vi "DSF.Engine.Framework.Active Plugins.vi"(8 "error in (no error)":errorcluster, 11 "Framework in":refnum<class "Framework.lvclass">) -> (0 "error out":errorcluster, 2 "active Plugin indices":i32[](array[numeric]), 3 "Framework out":refnum<class "Framework.lvclass">)   [LabVIEW 2016, in "DSF.Engine.lvlib" / "Framework.lvclass"]
uses:
  Framework.lvclass
  Framework.lvclass/Framework.ctl
  Plugin/Plugin.lvclass/Plugin.ctl
  Shared/Classes/Timing/DSF.Shared.Timing.lvclass
  Plugin/Plugin.lvclass
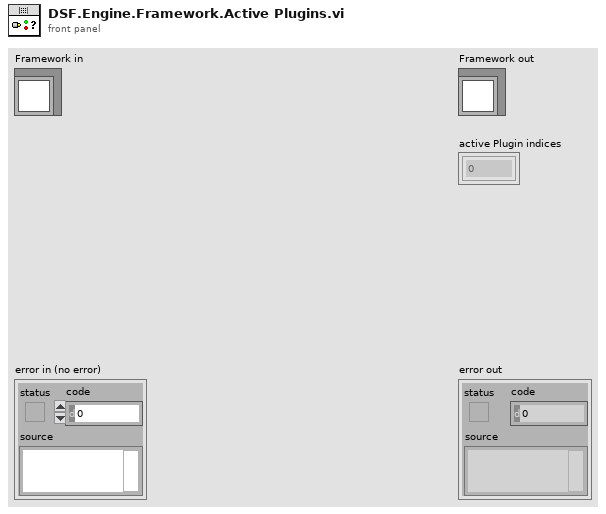
[diagram p1: front panel]
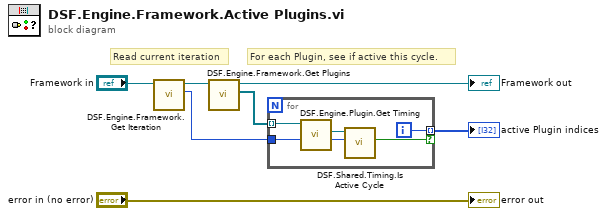
[diagram p0: block diagram]
diagram:
  # "For each Plugin, see if active this cycle."
  # "Read current iteration"
  n1 = call "DSF.Engine.Framework.Get Iteration.vi"("Framework in"="Framework in") -> ("iteration"=w4:u64, "Framework out"=w5:refnum<class "Framework.lvclass">)  [unwired: 9 in]
  n2 = call "DSF.Engine.Framework.Get Plugins.vi"("Framework in"=w5) -> ("Plugins"=w7:refnum<class "Plugin.lvclass">[], "Framework out"=→"Framework out":refnum<class "Framework.lvclass">)  [unwired: 9 in]
  n3 = for {
    tunnel: [w12] -> w3 mode=indexing if=w11
    tunnel: w7 -> [w9] mode=indexing
    tunnel: w4 -> [w8]
    i -> [w12]
    n4 = call "DSF.Engine.Plugin.Get Timing.vi"("Plugin in"=w9) -> ("Timing"=w10:refnum<class "DSF.Shared.Timing.lvclass">)  [unwired: 9 in, 1 out]
    n5 = call "DSF.Shared.Timing.Is Active Cycle.vi"("iteration"=w8, "Timing in"=w10) -> ("active?"=w11:bool)  [unwired: 8 in, 1 out]
  }
  "active Plugin indices" <- w3
  "error out" <- "error in (no error)"
